vi "e.gate Example - Real Time Clock.vi"() -> ()   [LabVIEW 2016]
uses:
  e.gate Protocol Type.ctl
  e.gate Time.ctl
panel:
  in  "Stopp":bool
  out "New Time":T1
  in  "Offset":T1
  out "Actual Time":T1
  out "error out":errorcluster
  in  "Enable writing":bool
  in  "Protocol":T2
  in  "IP Address":string
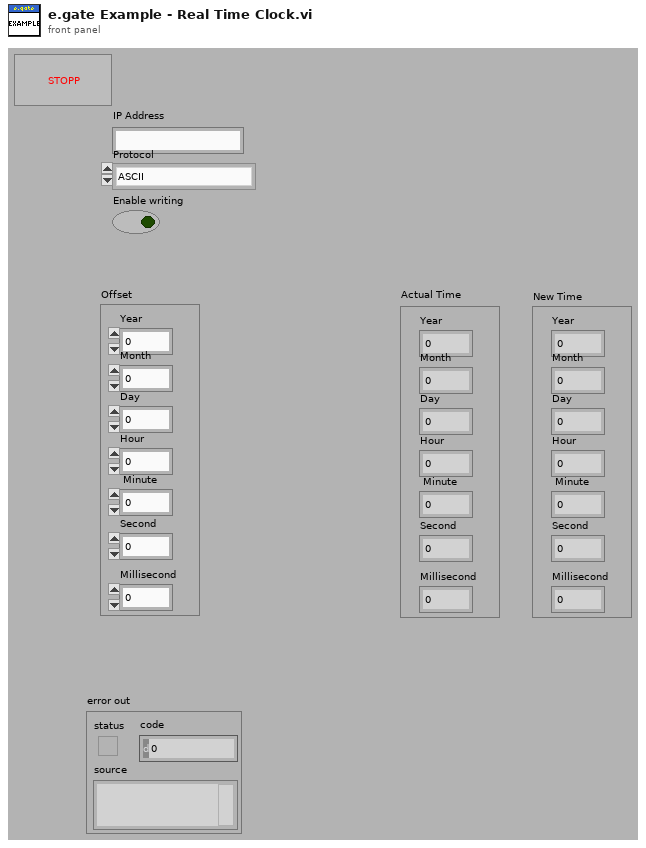
[diagram p1: front panel]
types:
  T1 = typedef "e.gate Time.ctl" = cluster{"Year":dbl, "Month":dbl, "Day":dbl, "Hour":dbl, " Minute":dbl, "Second":dbl, "Millisecond":dbl}
  T2 = typedef "e.gate Protocol Type.ctl" = enum16{"ASCII", "HighspeedPort Online", "HighspeedPort Buffer", "eGateHighspeedPortDLL "}
  T3 = typedef "e.gate Configuration.ctl" = cluster{"connection ID":refnum<k5>, "IPAddress":string, "BufferIndex":i32, "StateMessage":string, "StateCode":i8, "HeaderSize":i32, "BufferSize":i32, "IsBigEndian":i32, "Version":i32, "ChannelCount":i32, "FrameLength":i32, "StartTime":dbl, "dActTimeToSecondFactor":dbl, "StartTimeToDayFactor":dbl, "BufferFillRate":dbl, "SampleRate":dbl, "ChannelData":T4[], "DecodeTimeFormat":string, "SummaryPath":string, "WithCheckSum":i32, "dActTimeDataType":T5, "MaxWriteCount":i32, "MaxReadCount":i32, "TempOffsetRead":i32, "TempLengthRead":i32, "Protocol":T2, "IsSupported":i32, "InputAccessList":i32[], "OutputAccessList":i32[], "DataSource":enum16{"CircleBuffer", "test.con Logger", "test.con Archive"}, "Modules":T6[], "DLL-Handle":T7}
  T4 = typedef "e.gate Channel Data.ctl" = cluster{"VariableName":string, "DataDirection":string, "DataType":string, "DataTypeIndex":T5, "Precision":i16, "FieldLengtht":i16, "ByteCount":i32, "Format":string, "Unit":string, "InputAccessOffset":i32, "OutputAccessOffset":i16, "InputAccessIndex":i16, "OutputAccessIndex":i16, "VarType":string}
  T5 = typedef "e.gate Data Type.ctl" = enum16{"NO", "BOOL", "SINT8", "USINT8", "SINT16", "USINT16", "SINT32", "USINT32", "FLOAT", "SET8", "SET16", "SET32", "DOUBLE", "SINT64", "USINT64", "SET64"}
  T6 = typedef "e.gate Module  Data.ctl" = cluster{"Type":string, "Location":string, "VariablesCount":i16, "UartIndex":i16, "Address":i16, "SystemOffset":i16}
  T7 = typedef "e.gateHSP_DLLhandle.ctl" = cluster{"clientInstance":i32, "connectionInstance":i32}
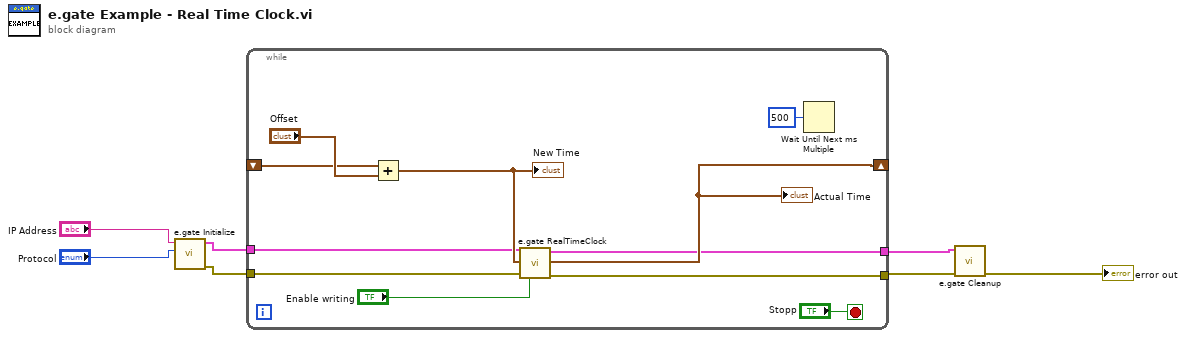
[diagram p0: block diagram]
diagram:
  n1 = call "e.gate Initialize.vi"("Protocol"="Protocol", "IP Address"="IP Address") -> ("error out"=w4:errorcluster, "e.gate Configuration"=w5:T3)  [unwired: 2 in, 6 out]
  n2 = while {
    tunnel: [w7] -> w6
    shift-right: [w14] -> _
    shift-left: _ -> [w13]
    tunnel: w5 -> [w10]
    tunnel: w4 -> [w9]
    tunnel: [w8] -> w1
    stop <- "Stopp" stop-if-true
    n3 = Add(x=w13, y="Offset") -> (x+y=w12:T1)
    "New Time" <- w12
    n4 = call "e.gate RealTimeClock.vi"("Configuration  in"=w10, "e.gate Time in"=w12, "error in (no error)"=w9, "Enable writing"="Enable writing") -> ("Configuration out"=w8:T3, "e.gate Time out"=w14:T1, "error out"=w7:errorcluster)  [unwired: 21 out]
    "Actual Time" <- w14
    n5 = Wait Until Next ms Multiple(millisecond multiple=u32 500 ("Vielfache von ms")) -> ()  [unwired: 1 out]
  }
  "error out" <- w6
  n6 = call "e.gate Cleanup.vi"("e.gate Configuration"=w1) -> ()  [unwired: 1 in, 10 out]
